vi "OAT Map to  RPM.vi"(5 "RPM indices":i32[](array[numeric]), 6 "RPM boundaries":i32[](array[numeric]), 7 "energy level in ranges":dbl[](array[numeric]) format="%.2f") -> (3 "energy level at RPMs":dbl[](array[numeric]) format="%.2f")   [LabVIEW 2017, in "SoundVib_Gabor.lvlib"]
uses:
  <vilib>/addons/Sound and Vibration/Order Analysis/Gabor Order Tracking/SoundVib_Gabor.lvlib
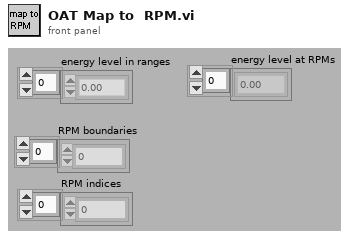
[diagram p1: front panel]
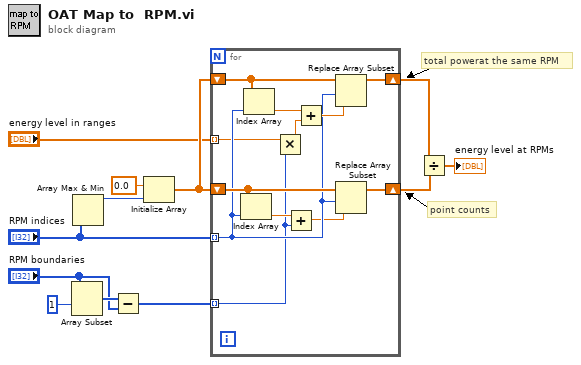
[diagram p0: block diagram]
diagram:
  # "point counts"
  # "total powerat the same RPM"
  n1 = Array Subset(array="RPM boundaries", index=1) -> (w12:i32[])  [unwired: 1 in]
  n2 = Array Max & Min(array="RPM indices") -> (max value=w1:i32)  [unwired: 3 out]
  n3 = Subtract(x=w12, y="RPM boundaries") -> (x-y=w9:i32[])
  n4 = Initialize Array(0.0, w1) -> (w7:dbl[])
  n5 = for {
    tunnel: "RPM indices" -> [w18] mode=indexing
    tunnel: "energy level in ranges" -> [w13] mode=indexing
    tunnel: w9 -> [w15] mode=indexing
    shift-right: [w23] -> w6
    shift-left: w7 -> [w24]
    shift-right: [w20] -> w5
    shift-left: w7 -> [w19]
    n6 = Index Array(array=w19, index=w18) -> (element=w17:dbl)
    n7 = Index Array(array=w24, index=w18) -> (element=w22:dbl)
    n8 = Multiply(x=w13, y=w15) -> (x*y=w14:dbl)
    n9 = Add(x=w17, y=w15) -> (x+y=w16:dbl)
    n10 = Add(x=w22, y=w14) -> (x+y=w21:dbl)
    n11 = Replace Array Subset(array=w24, new element=w21, index=w18) -> (w23:dbl[])
    n12 = Replace Array Subset(array=w19, new element=w16, index=w18) -> (w20:dbl[])
  }
  n13 = Divide(x=w6, y=w5) -> (x/y=→"energy level at RPMs":dbl[])
